vi "Read Weekly DoW.vi"(8 "error in (no error)":errorcluster, 11 "Weekly in":refnum<class "Weekly.lvclass">) -> (0 "error out":errorcluster, 2 "Weekly DoW":T1 caption="DoW", 3 "Weekly out":refnum<class "Weekly.lvclass">)   [LabVIEW 2020, in "Weekly.lvclass"]
uses:
  Weekly.lvclass
  Weekly.lvclass/Weekly.ctl
  Day of the Week STYP.ctl
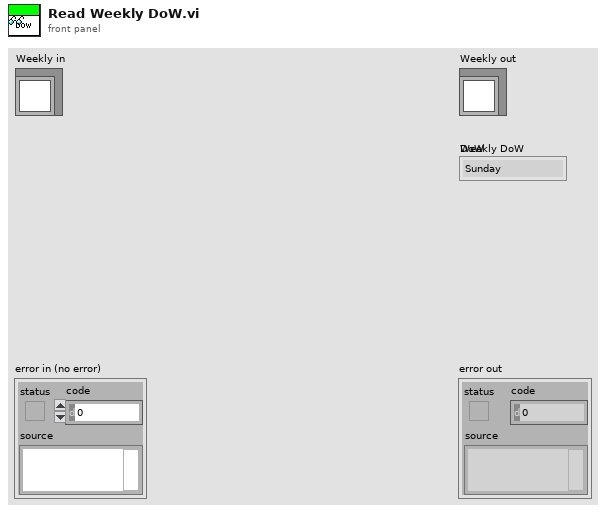
[diagram p1: front panel]
types:
  T1 = typedef "Day of the Week STYP.ctl" = enum16{"Sunday", "Monday", "Tuesday", "Wednesday", "Thursday", "Friday", "Saturday"}
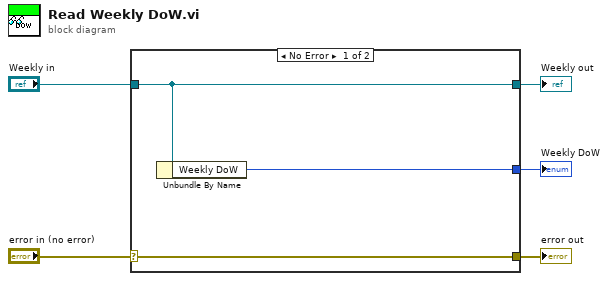
[diagram p0: block diagram]
diagram:
  n1 = case shown="No Error" "error in (no error)" {
    selector: "error in (no error)" -> [w8 w9]
    tunnel: [w8 w9] -> w4
    tunnel: [w7 w10] -> w2
    tunnel: "Weekly in" -> [w7 w10]
    tunnel: [w6 _] -> w1
    frame No Error {
      n2 = Unbundle By Name(w7) -> ("Weekly DoW"=w6:T1)
    }
    frame Error {
    }
  }
  "error out" <- w4
  "Weekly out" <- w2
  "Weekly DoW" <- w1
